vi "current measur.vi"() -> ()   [LabVIEW 2019]
uses:
  <vilib>/DAQmx/read.llb/DAQmx Read (Analog DBL 1Chan 1Samp).vi
  <vilib>/DAQmx/miscellaneous.llb/DAQmx Fill In Error Info.vi
panel:
  out "Amp":dbl format="%0.2f"
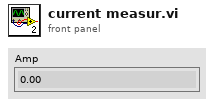
[diagram p1: front panel]
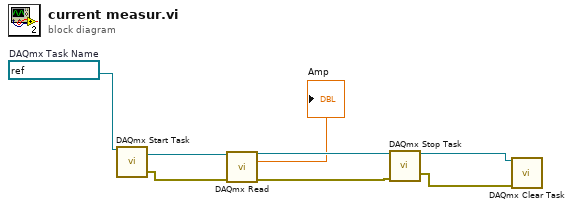
[diagram p0: block diagram]
diagram:
  w1 = refnum<k21> "CurrentTask"  # DAQmx Task Name
  n1 = call <vilib>:"DAQmx Start Task.vi"("task/channels in"=w1) -> ("task out"=w8:refnum<k21>, "error out"=w7:errorcluster)  [unwired: 13 in]
  n2 = call-poly <vilib>:"DAQmx Read.vi"("task/channels in"=w8, "error in"=w7) -> ("task out"=w5:refnum<k21>, "data"=→"Amp":dbl, "error out"=w6:errorcluster)  [unwired: 11 in]
  n3 = call <vilib>:"DAQmx Stop Task.vi"("task/channels in"=w5, "error in"=w6) -> ("task out"=w4:refnum<k21>, "error out"=w3:errorcluster)  [unwired: 12 in]
  n4 = call <vilib>:"DAQmx Clear Task.vi"("task in"=w4, "error in"=w3) -> ()  [unwired: 13 in, 1 out]
